vi "GetItems.vi"(8 "Error In":errorcluster, 11 "reference in":refnum<class "DinnerMenu.lvclass">) -> (0 "Error Out":errorcluster, 2 "Items":refnum<class "IEnumerable.lvclass">, 3 "reference out":refnum<class "DinnerMenu.lvclass">)   [LabVIEW 2020, in "DinnerMenu.lvclass"]
uses:
  DinnerMenu.lvclass
  IEnumerable_interface/IEnumerable.lvclass
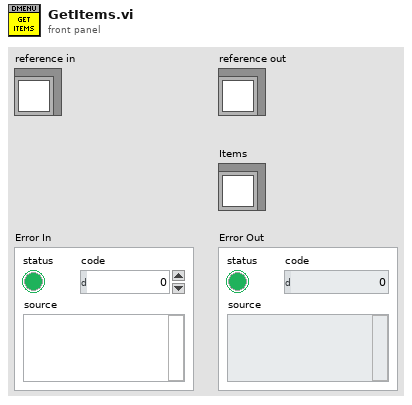
[diagram p1: front panel]
types:
  T1 = typedef "DinnerMenu.lvclass/ObjectAttributes.ctl" = cluster{"Max":i32, "_count":i32, "_items":refnum<class "Menu.lvclass">[], "Items":refnum<class "IEnumerable.lvclass">}
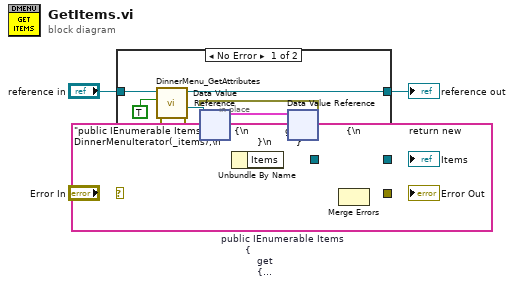
[diagram p0: block diagram]
diagram:
  (unwired) "public IEnumerable Items\n        {\n            get\n            {\n                return new DinnerMenuIterator(_items);\n            }\n        }"  # public IEnumerable Items         {             get             {                 return new DinnerMenuIterator(_items);             }         }
  n1 = case shown="No Error" "Error In" {
    selector: "Error In" -> [w14 w18]
    tunnel: [w12 w18] -> w4
    tunnel: [w9 w17] -> w2
    tunnel: "reference in" -> [w10 w17]
    tunnel: [w6 _] -> w1
    frame No Error {
      n2 = call "DinnerMenu_GetAttributes.vi"("error in (no error)"=w14, "OnlyGetDvrReference(False)"=TRUE, "reference in"=w10) -> ("error out"=w13:errorcluster, "DataRef"=w7:refnum<data-value>, "reference out"=w9:refnum<class "DinnerMenu.lvclass">)  [unwired: 5 in, 1 out]
      n3 = in-place {
        in-place-border: [w16] -> w6
        n4 = in-place-dvr #1(w7) -> (w15:T1)  [unwired: 1 out]
        n5 = Unbundle By Name(w15) -> ("Items"=w16:refnum<class "IEnumerable.lvclass">)
        n6 = in-place-dvr #1(w15) -> (w11:errorcluster)  [unwired: 1 out]
      }
      n7 = Merge Errors(w13, w11) -> (w12:errorcluster)
    }
    frame Error {
    }
  }
  "Error Out" <- w4
  "reference out" <- w2
  "Items" <- w1
